vi "E-Series Reader.vi"(8 "error in":errorcluster, 11 "E-Series File Names":T2) -> (0 "error out":errorcluster, 3 "E-Series Data":T1)   [LabVIEW 2018, in "E-Series Reader.lvlib"]
doc: "Loads the E-Series data from the CSV files specified by <b>E-Series File Names</b>.\n\nThe VI receives an array of E-Series file names and an <b>error in</b> status. It reads the corresponding CSV files and returns the loaded E-Series values in <b>E-Series Data</b>, together with the resulting <b>error out</b> status."
uses:
  E-Series Reader.lvlib
  E-Series File Names--array.ctl
  Series Data--cluster.ctl
  States--enum.ctl
  E-Series Index--enum.ctl
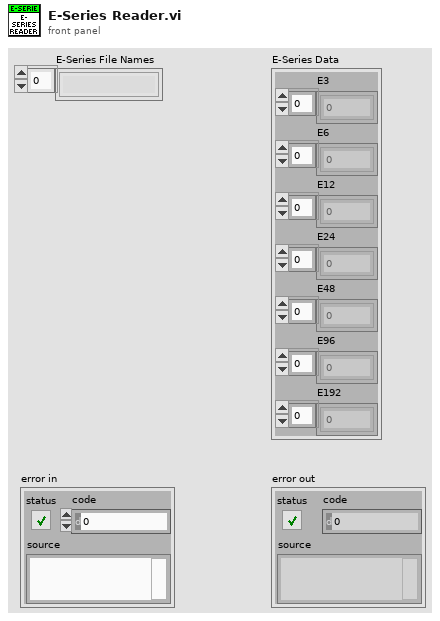
[diagram p1: front panel]
types:
  T1 = typedef "E-Series Reader.lvlib/series data--cluster.ctl" = cluster{"E3":u16[], "E6":u16[], "E12":u16[], "E24":u16[], "E48":u16[], "E96":u16[], "E192":u16[]}
  T2 = typedef "E-Series Reader.lvlib/e-series file names--array.ctl" = string[]
  T3 = typedef "E-Series Reader.lvlib/states--enum.ctl" = enum16{"Initialize", "Read E3 Series", "Read E6 Series", "Read E12 Series", "Read E24 Series", "Read E48 Series", "Read E96 Series", "Read E192 Series", "Error", "Shutdown"}
  T4 = typedef "E-Series Reader.lvlib/e-series index--enum.ctl" = enum32{"E3 Series", "E6 Series", "E12 Series", "E24 Series", "E48 Series", "E96 Series", "E192 Series"}
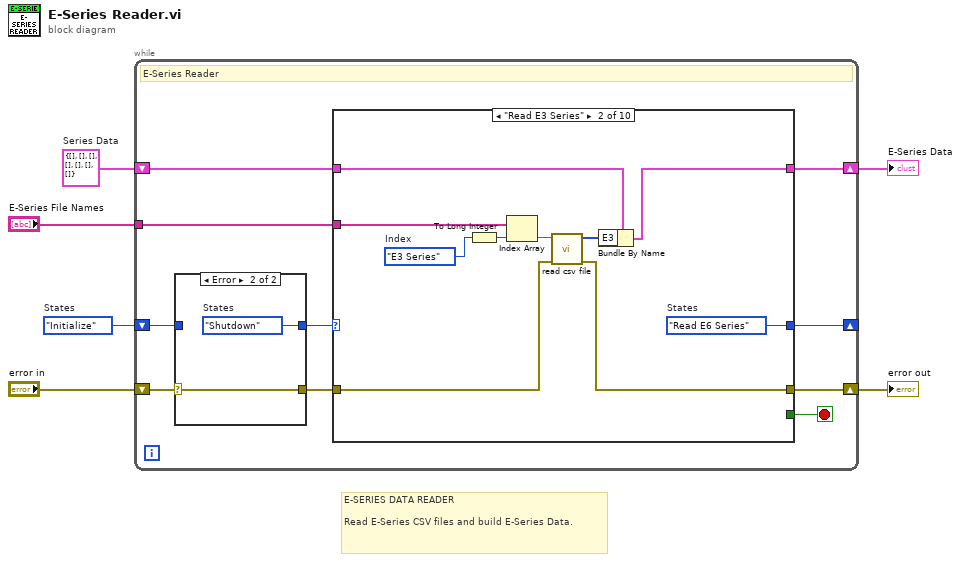
[diagram p0: block diagram]
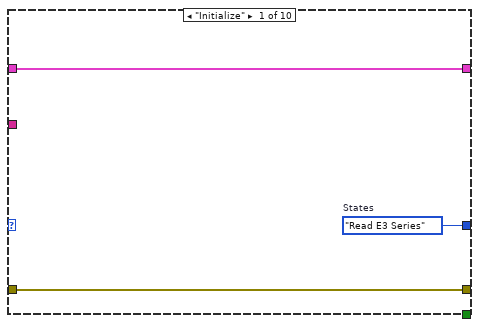
[diagram p3: hidden frame]
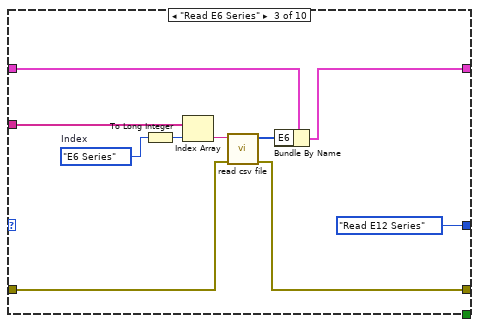
[diagram p4: hidden frame]
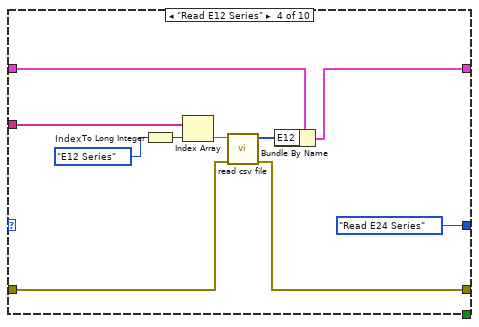
[diagram p5: hidden frame]
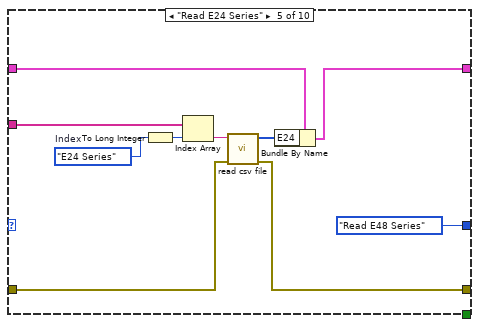
[diagram p6: hidden frame]
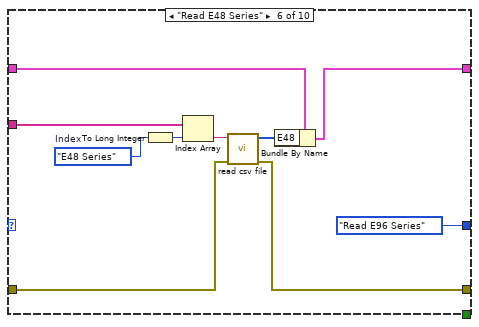
[diagram p7: hidden frame]
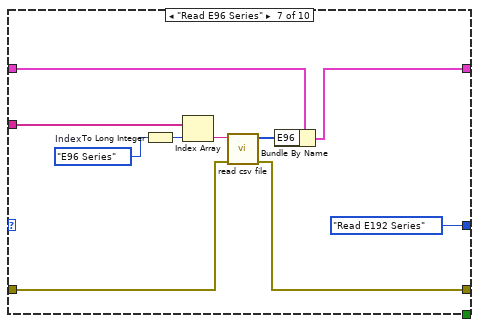
[diagram p8: hidden frame]
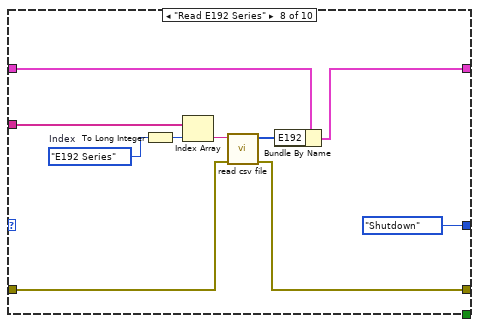
[diagram p9: hidden frame]
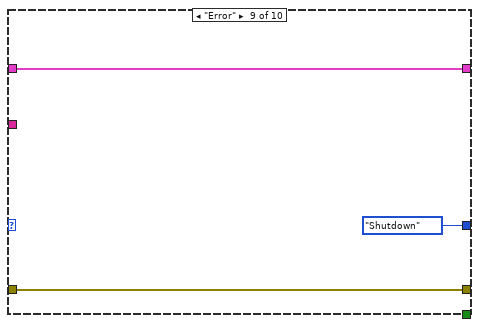
[diagram p10: hidden frame]
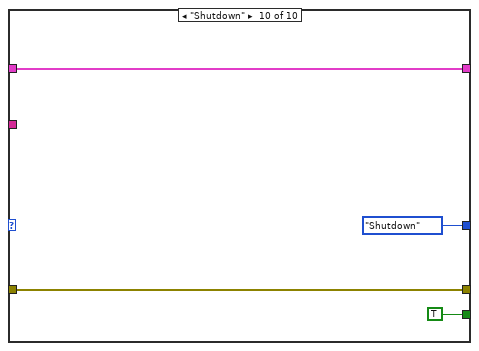
[diagram p11: hidden frame]
diagram:
  w3 = T1 {"E3"=[], "E6"=[], "E12"=[], "E24"=[], "E48"=[], "E96"=[], "E192"=[]}  # Series Data
  w6 = states--enum."Initialize"  # States
  # "E-SERIES DATA READER\n\nRead E-Series CSV files and build E-Series Data."
  n1 = while {
    shift-right: [w8] -> _
    shift-left: w6 -> [w16]
    shift-right: [w12] -> w5
    shift-left: "error in" -> [w15]
    shift-right: [w9] -> w1
    shift-left: w3 -> [w11]
    tunnel: "E-Series File Names" -> [w7]
    stop <- w10 stop-if-true
    # "E-Series Reader"
    n2 = case shown="Error" w15 {
      selector: w15 -> [w17 w20]
      tunnel: w16 -> [w18 _]
      tunnel: [w18 w19] -> w14
      tunnel: [w17 w20] -> w13
      frame No Error {
      }
      frame Error {
        w19 = states--enum."Shutdown"  # States
      }
    }
    n3 = case shown="\"Read E3 Series\"" w14 {
      tunnel: w13 -> [w23 w31 w41 w51 w62 w71 w81 w91 w94 w100]
      tunnel: [w23 w30 w40 w50 w61 w70 w80 w90 w94 w100] -> w12
      tunnel: w11 -> [w22 w33 w43 w53 w60 w73 w83 w93 w96 w99]
      tunnel: [w22 w32 w42 w52 w59 w72 w82 w92 w96 w99] -> w9
      tunnel: [_ _ _ _ _ _ _ _ _ TRUE] -> w10
      tunnel: [w21 w28 states--enum."Read E12 Series" ("States") states--enum."Read E24 Series" ("States") states--enum."Read E48 Series" ("States") states--enum."Read E96 Series" ("States") states--enum."Read E192 Series" ("States") states--enum."Shutdown" ("States") states--enum."Shutdown" ("States") states--enum."Shutdown" ("States")] -> w8
      tunnel: w7 -> [_ w27 w35 w45 w55 w65 w75 w85 _ _]
      frame "Initialize" {
        w21 = states--enum."Read E3 Series"  # States
      }
      frame "Read E3 Series" {
        w26 = e-series_index--enum."E3 Series"  # Index
        w28 = states--enum."Read E6 Series"  # States
        n4 = To Long Integer(number=w26) -> (32bit integer=w25:i32)
        n5 = Index Array(array=w27, index=w25) -> (element=w24:string)
        n6 = call "read csv file.vi"("error in (no error)"=w31, "File name"=w24) -> ("error out"=w30:errorcluster, "Series"=w29:u16[])  [unwired: 8 in]
        n7 = Bundle By Name(cluster=w33, "E3"=w29) -> (w32:T1)
      }
      frame "Read E6 Series" {
        w37 = e-series_index--enum."E6 Series"  # Index
        n8 = To Long Integer(number=w37) -> (32bit integer=w36:i32)
        n9 = Index Array(array=w35, index=w36) -> (element=w34:string)
        n10 = call "read csv file.vi"("error in (no error)"=w41, "File name"=w34) -> ("error out"=w40:errorcluster, "Series"=w39:u16[])  [unwired: 8 in]
        n11 = Bundle By Name(cluster=w43, "E6"=w39) -> (w42:T1)
      }
      frame "Read E12 Series" {
        w47 = e-series_index--enum."E12 Series"  # Index
        n12 = To Long Integer(number=w47) -> (32bit integer=w46:i32)
        n13 = Index Array(array=w45, index=w46) -> (element=w44:string)
        n14 = call "read csv file.vi"("error in (no error)"=w51, "File name"=w44) -> ("error out"=w50:errorcluster, "Series"=w49:u16[])  [unwired: 8 in]
        n15 = Bundle By Name(cluster=w53, "E12"=w49) -> (w52:T1)
      }
      frame "Read E24 Series" {
        w57 = e-series_index--enum."E24 Series"  # Index
        n16 = To Long Integer(number=w57) -> (32bit integer=w56:i32)
        n17 = Index Array(array=w55, index=w56) -> (element=w54:string)
        n18 = call "read csv file.vi"("error in (no error)"=w62, "File name"=w54) -> ("error out"=w61:errorcluster, "Series"=w63:u16[])  [unwired: 8 in]
        n19 = Bundle By Name(cluster=w60, "E24"=w63) -> (w59:T1)
      }
      frame "Read E48 Series" {
        w67 = e-series_index--enum."E48 Series"  # Index
        n20 = To Long Integer(number=w67) -> (32bit integer=w66:i32)
        n21 = Index Array(array=w65, index=w66) -> (element=w64:string)
        n22 = call "read csv file.vi"("error in (no error)"=w71, "File name"=w64) -> ("error out"=w70:errorcluster, "Series"=w69:u16[])  [unwired: 8 in]
        n23 = Bundle By Name(cluster=w73, "E48"=w69) -> (w72:T1)
      }
      frame "Read E96 Series" {
        w77 = e-series_index--enum."E96 Series"  # Index
        n24 = To Long Integer(number=w77) -> (32bit integer=w76:i32)
        n25 = Index Array(array=w75, index=w76) -> (element=w74:string)
        n26 = call "read csv file.vi"("error in (no error)"=w81, "File name"=w74) -> ("error out"=w80:errorcluster, "Series"=w79:u16[])  [unwired: 8 in]
        n27 = Bundle By Name(cluster=w83, "E96"=w79) -> (w82:T1)
      }
      frame "Read E192 Series" {
        w87 = e-series_index--enum."E192 Series"  # Index
        n28 = To Long Integer(number=w87) -> (32bit integer=w86:i32)
        n29 = Index Array(array=w85, index=w86) -> (element=w84:string)
        n30 = call "read csv file.vi"("error in (no error)"=w91, "File name"=w84) -> ("error out"=w90:errorcluster, "Series"=w89:u16[])  [unwired: 8 in]
        n31 = Bundle By Name(cluster=w93, "E192"=w89) -> (w92:T1)
      }
      frame "Error" {
      }
      frame "Shutdown" {
      }
    }
  }
  "error out" <- w5
  "E-Series Data" <- w1
